vi "process_document.vi"(0 "abstract_dataprocessing_base in":refnum<class "abstract_dataprocessing_base.lvclass">, 5 "documents":refnum<class "data_document.lvclass">[](array[class]), 11 "error in (no error)":errorcluster) -> (4 "abstract_dataprocessing_base out":refnum<class "abstract_dataprocessing_base.lvclass">, 6 "nodes":refnum<class "data_node.lvclass">[](array[class]), 15 "error out":errorcluster)   [LabVIEW 2020, in "abstract_dataprocessing_base.lvclass"]
uses:
  abstract_dataprocessing_base.lvclass
  data/data_document/data_document.lvclass
  data/data_node/data_node.lvclass
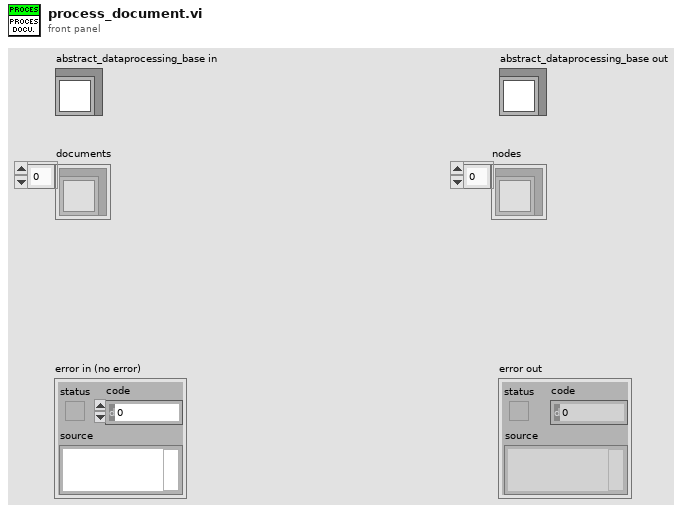
[diagram p1: front panel]
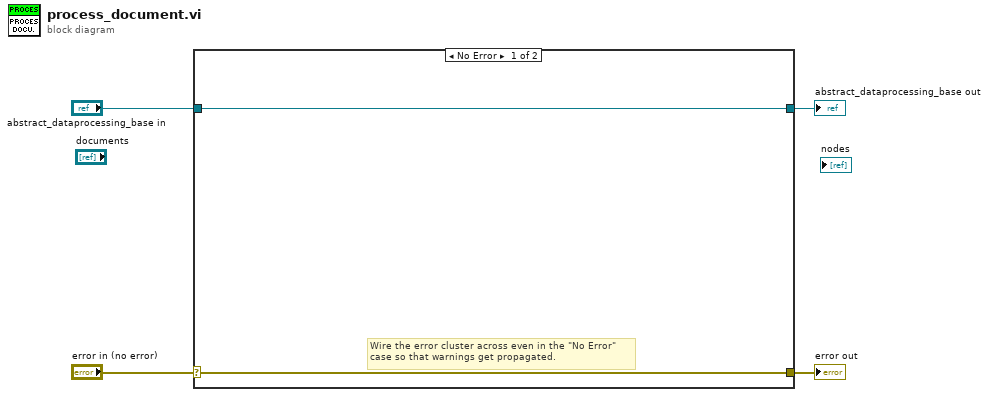
[diagram p0: block diagram]
diagram:
  n1 = case shown="No Error" "error in (no error)" {
    selector: "error in (no error)" -> [w5 w8]
    tunnel: [w5 w8] -> w3
    tunnel: [w6 w7] -> w1
    tunnel: "abstract_dataprocessing_base in" -> [w6 w7]
    frame No Error {
      # "Wire the error cluster across even in the \"No Error\"\ncase so that warnings get propagated."
    }
    frame Error {
    }
  }
  "error out" <- w3
  "abstract_dataprocessing_base out" <- w1
